vi "FTW-ActorRef-Initialize.vi"(0 "FTW Actor Reference":refnum<class "FTW-ActorReference.lvclass">, 5 "Actor VI Filepath":path, 7 "Actor Configuration":variant, 9 "Actor Context":refnum<class "FTW-Actor-Context.lvclass">, 11 "error in":errorcluster) -> (4 "FTW Actor Reference out":refnum<class "FTW-ActorReference.lvclass">, 15 "error out":errorcluster)   [LabVIEW 2014, in "FTW-ActorReference.lvclass"]
uses:
  FTW-ActorReference.lvclass
  Context/FTW-Actor-Context.lvclass
panel:
  # "Inputs"
  # "Outputs"
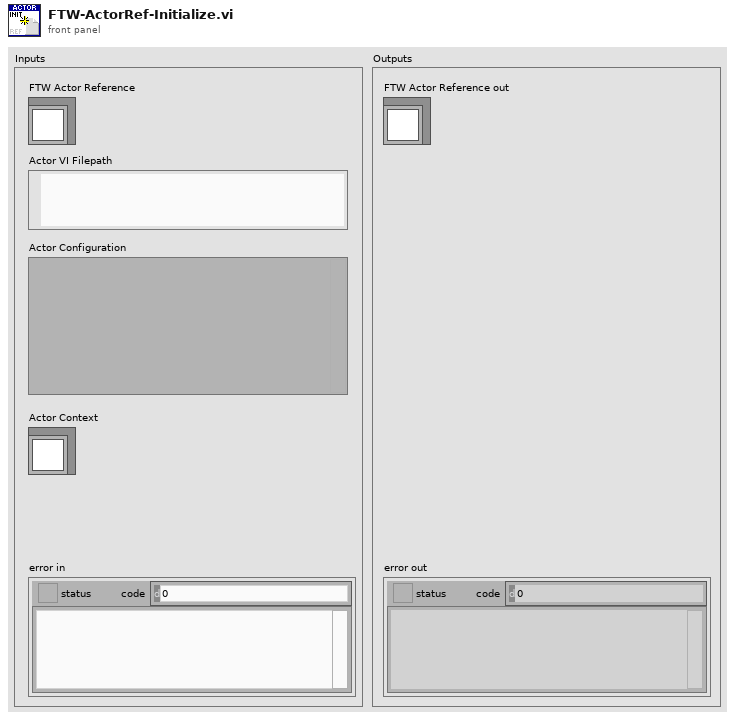
[diagram p1: front panel]
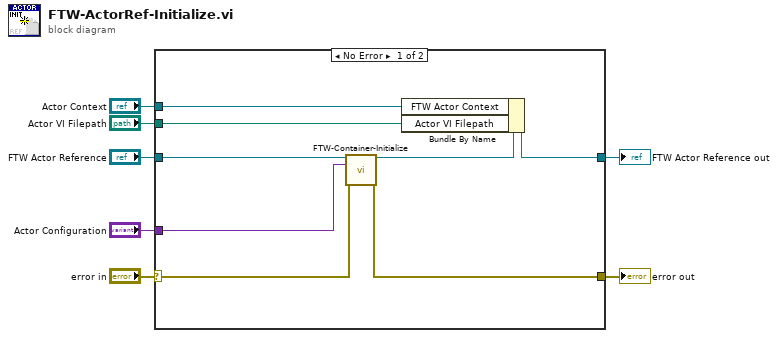
[diagram p0: block diagram]
diagram:
  n1 = case shown="No Error" "error in" {
    selector: "error in" -> [w11 w17]
    tunnel: [w10 w17] -> w6
    tunnel: "FTW Actor Reference" -> [w13 w16]
    tunnel: [w15 w16] -> w4
    tunnel: "Actor VI Filepath" -> [w14 _]
    tunnel: "Actor Configuration" -> [w9 _]
    tunnel: "Actor Context" -> [w8 _]
    frame No Error {
      n2 = call-dynamic "FTW-Container-Initialize.vi"("Container"=w13, "LabVIEW Data Structure"=w9, "error in"=w11) -> ("Container out"=w12:refnum<class "FTW-ActorReference.lvclass">, "error out"=w10:errorcluster)  [unwired: 11 in]
      n3 = Bundle By Name(cluster=w12, "FTW Actor Context"=w8, "Actor VI Filepath"=w14) -> (w15:refnum<class "FTW-ActorReference.lvclass">)
    }
    frame Error {
    }
  }
  "error out" <- w6
  "FTW Actor Reference out" <- w4
